vi "Decrement Score.vi"(8 "error in (no error)":errorcluster, 10 "Points Lost":i32, 11 "Contestant in":refnum<class "Contestant.lvclass">) -> (0 "error out":errorcluster, 3 "Contestant out":refnum<class "Contestant.lvclass">)   [LabVIEW 2024, in "Contestant.lvlib" / "Contestant.lvclass"]
uses:
  Contestant.lvclass
  Contestant.lvclass/Contestant.ctl
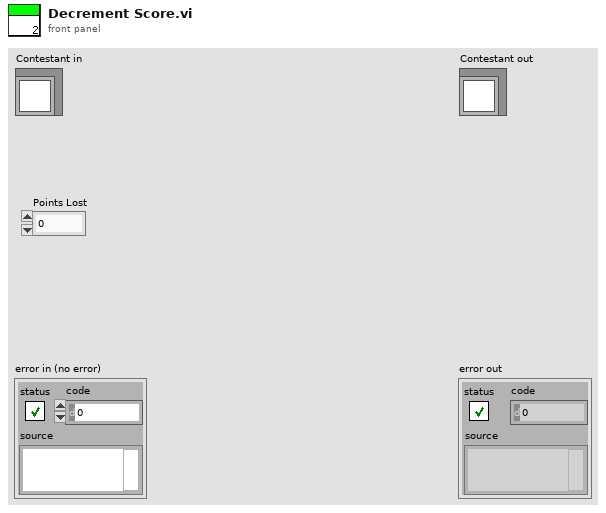
[diagram p1: front panel]
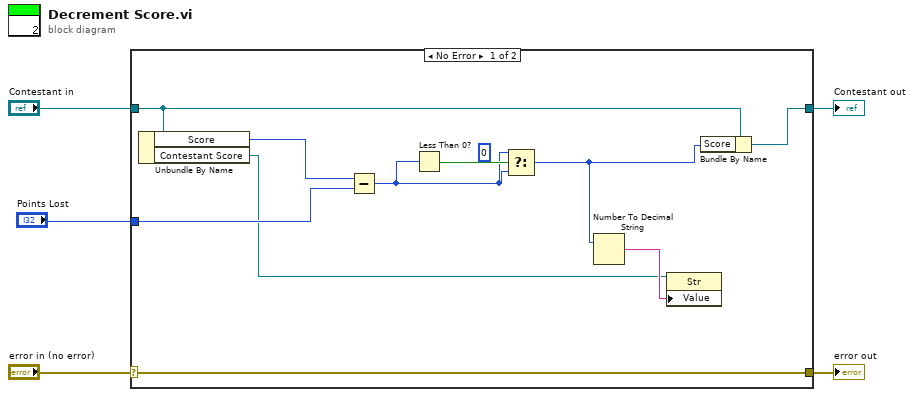
[diagram p0: block diagram]
diagram:
  n1 = case shown="No Error" "error in (no error)" {
    selector: "error in (no error)" -> [w15 w17]
    tunnel: [w15 w17] -> w4
    tunnel: [w13 w16] -> w2
    tunnel: "Contestant in" -> [w14 w16]
    tunnel: "Points Lost" -> [w11 _]
    frame No Error {
      (unwired) 0 ("t")
      n2 = Unbundle By Name(w14) -> ("Score"=w12:i32, "Contestant Score"=w8:refnum<vi>)
      n3 = Subtract(x=w12, y=w11) -> (x-y=w6:i32)
      n4 = Less Than 0?(x=w6) -> (x < 0?=w10:bool)
      n5 = Select(t=w6, s=w10, f=w6) -> (s? t:f=w7:i32)
      n6 = Number To Decimal String(number=w7) -> (decimal integer string=w9:string)  [unwired: 1 in]
      n7 = property class="Str"(reference=w8, "Value"=w9) -> ()  [unwired: 1 in, 2 out]
      n8 = Bundle By Name(cluster=w14, "Score"=w7) -> (w13:refnum<class "Contestant.lvclass">)
    }
    frame Error {
    }
  }
  "error out" <- w4
  "Contestant out" <- w2
